vi "SCTL Sector Accumulation Pipelined V2.vi"() -> (3 "New Data?":bool)   [LabVIEW 2013]
uses:
  <vilib>/rvi/FIFO/Fifo_Resource/nirvififoEmulationReadFpgaImpl.vi
  <vilib>/rvi/DataTransferAndStorage/Container/Common/niFpgaContainerGetUniqueNameForEmu.vi
  <vilib>/rvi/Memory/Memory_Emulation/nirvimemoryFastEmulationFpgaImpl.vi
  <instcachedir>/0/nirvimemoryFastEmulationFpgaImpl_5FBAB50466BC4C939F684F8805638BFC.lvgen/nirvimemoryFastEmulationFpgaImpl_5FBAB50466BC4C939F684F8805638BFC_011.vi
  <vilib>/rvi/Memory/Memory_Emulation/nirvimemoryFastEmulation.vi
  <vilib>/rvi/Memory/Memory_Emulation/nirvimemoryEmulation.vi
  <vilib>/rvi/DataTransferAndStorage/Container/XNode/niFpgaContainer.xnode
  <vilib>/rvi/FIFO/Fifo_Resource/nirvififoEmulationRead.vi
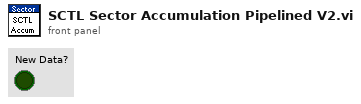
[diagram p1: front panel]
types:
  T1 = cluster{"Accumulated Intensity":u32, "Count":u16}
  T2 = cluster{"Accumulated Intensity":u32, "Count":u16}[]
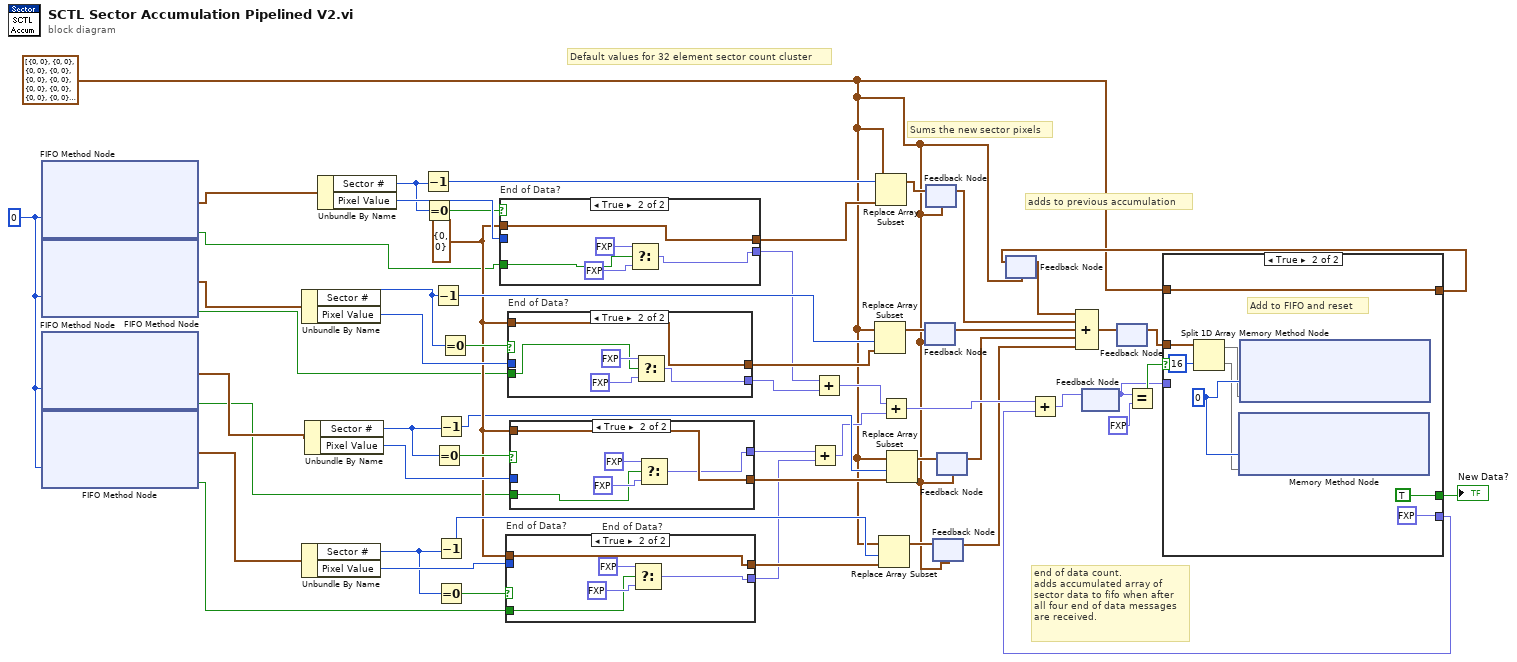
[diagram p0: block diagram]
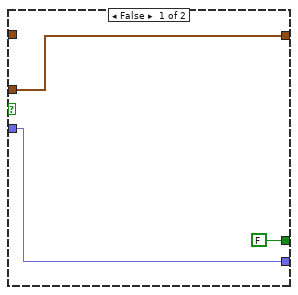
[diagram p2: hidden frame]
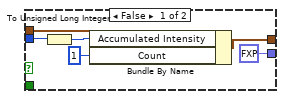
[diagram p3: hidden frame]
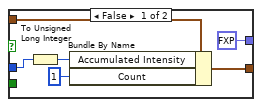
[diagram p4: hidden frame]
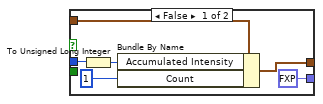
[diagram p5: hidden frame]
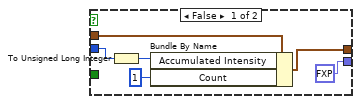
[diagram p6: hidden frame]
diagram:
  w32 = T1 {"Accumulated Intensity"=0, "Count"=0} ("Accumulated Sector Cluster")
  w1 = T2 [{"Accumulated Intensity"=0, "Count"=0}, {"Accumulated Intensity"=0, "Count"=0}, {"Accumulated Intensity"=0, "Count"=0}, {"Accumulated Intensity"=0, "Count"=0}, {"Accumulated Intensity"=0, "Count"=0}, {"Accumulated Intensity"=0, "Count"=0}, {"Accumulated Intensity"=0, "Count"=0}, {"Accumulated Intensity"=0, "Count"=0}, {"Accumulated Intensity"=0, "Count"=0}, {"Accumulated Intensity"=0, "Count"=0}, {"Accumulated Intensity"=0, "Count"=0}, {"Accumulated Intensity"=0, "Count"=0}, {"Accumulated Intensity"=0, "Count"=0}, {"Accumulated Intensity"=0, "Count"=0}, {"Accumulated Intensity"=0, "Count"=0}, {"Accumulated Intensity"=0, "Count"=0}, {"Accumulated Intensity"=0, "Count"=0}, {"Accumulated Intensity"=0, "Count"=0}, {"Accumulated Intensity"=0, "Count"=0}, {"Accumulated Intensity"=0, "Count"=0}, {"Accumulated Intensity"=0, "Count"=0}, {"Accumulated Intensity"=0, "Count"=0}, {"Accumulated Intensity"=0, "Count"=0}, {"Accumulated Intensity"=0, "Count"=0}, {"Accumulated Intensity"=0, "Count"=0}, {"Accumulated Intensity"=0, "Count"=0}, {"Accumulated Intensity"=0, "Count"=0}, {"Accumulated Intensity"=0, "Count"=0}, {"Accumulated Intensity"=0, "Count"=0}, {"Accumulated Intensity"=0, "Count"=0}, {"Accumulated Intensity"=0, "Count"=0}, {"Accumulated Intensity"=0, "Count"=0}] ("Data")
  w56 = 0 ("Timeout")
  # "end of data count.\nadds accumulated array of\nsector data to fifo when after\nall four end of data messages\nare received."
  # "adds to previous accumulation"
  # "Sums the new sector pixels"
  # "Default values for 32 element sector count cluster"
  n1 = xnode ("FIFO Method Node")("Timeout"=w56) -> ("Element"=w28:cluster{"Sector #":u8, "Pixel Value":u8}, "Timed Out?"=w24:bool)  [unwired: 1 in, 1 out]
  n2 = xnode ("FIFO Method Node")("Timeout"=w56) -> ("Element"=w27:cluster{"Sector #":u8, "Pixel Value":u8}, "Timed Out?"=w23:bool)  [unwired: 1 in, 1 out]
  n3 = xnode ("FIFO Method Node")("Timeout"=w56) -> ("Element"=w26:cluster{"Sector #":u8, "Pixel Value":u8}, "Timed Out?"=w22:bool)  [unwired: 1 in, 1 out]
  n4 = xnode ("FIFO Method Node")("Timeout"=w56) -> ("Element"=w25:cluster{"Sector #":u8, "Pixel Value":u8}, "Timed Out?"=w21:bool)  [unwired: 1 in, 1 out]
  n5 = Unbundle By Name(w27) -> ("Sector #"=w42:u8, "Pixel Value"=w52:u8)
  n6 = Unbundle By Name(w25) -> ("Sector #"=w38:u8, "Pixel Value"=w46:u8)
  n7 = Unbundle By Name(w26) -> ("Sector #"=w40:u8, "Pixel Value"=w49:u8)
  n8 = Unbundle By Name(w28) -> ("Sector #"=w44:u8, "Pixel Value"=w54:u8)
  n9 = Decrement(x=w44) -> (x-1=w55:u8)
  n10 = Equal To 0?(x=w44) -> (x = 0?=w43:bool)
  n11 = Decrement(x=w42) -> (x-1=w51:u8)
  n12 = Equal To 0?(x=w40) -> (x = 0?=w39:bool)
  n13 = Decrement(x=w40) -> (x-1=w30:u8)
  n14 = Decrement(x=w38) -> (x-1=w48:u8)
  n15 = Equal To 0?(x=w38) -> (x = 0?=w37:bool)
  n16 = Equal To 0?(x=w42) -> (x = 0?=w41:bool)
  n17 = case "End of Data?" shown="True" w43 {
    tunnel: w54 -> [w58 _]
    tunnel: [w62 w67] -> w53
    tunnel: w32 -> [w61 w67]
    tunnel: [fxp<+,1,1> 0.0 w63] -> w20
    tunnel: w24 -> [_ w66]
    frame False {
      n18 = To Unsigned Long Integer(number=w58) -> (unsigned 32bit integer=w57:u32)
      n19 = Bundle By Name(cluster=w61, "Accumulated Intensity"=w57, "Count"=u16 1) -> (w62:T1)
    }
    frame True {
      n20 = Select(t=fxp<+,1,1> 0.0, s=w66, f=fxp<+,1,1> 1.0) -> (s? t:f=w63:fxp<+,1,1>)
    }
  }
  n21 = case "End of Data?" shown="True" w37 {
    tunnel: [w73 w78] -> w47
    tunnel: w32 -> [w72 w78]
    tunnel: w46 -> [w69 _]
    tunnel: [fxp<+,1,1> 0.0 w74] -> w17
    tunnel: w21 -> [_ w75]
    frame False {
      n22 = To Unsigned Long Integer(number=w69) -> (unsigned 32bit integer=w68:u32)
      n23 = Bundle By Name(cluster=w72, "Accumulated Intensity"=w68, "Count"=u16 1) -> (w73:T1)
    }
    frame True {
      n24 = Select(t=fxp<+,1,1> 0.0, s=w75, f=fxp<+,1,1> 1.0) -> (s? t:f=w74:fxp<+,1,1>)
    }
  }
  n25 = case "End of Data?" shown="True" w41 {
    tunnel: w52 -> [w80 _]
    tunnel: w32 -> [w84 w89]
    tunnel: [w83 w89] -> w45
    tunnel: [fxp<+,1,1> 0.0 w85] -> w19
    tunnel: w23 -> [_ w86]
    frame False {
      n26 = To Unsigned Long Integer(number=w80) -> (unsigned 32bit integer=w79:u32)
      n27 = Bundle By Name(cluster=w84, "Accumulated Intensity"=w79, "Count"=u16 1) -> (w83:T1)
    }
    frame True {
      n28 = Select(t=fxp<+,1,1> 0.0, s=w86, f=fxp<+,1,1> 1.0) -> (s? t:f=w85:fxp<+,1,1>)
    }
  }
  n29 = case "End of Data?" shown="True" w39 {
    tunnel: [w95 w100] -> w50
    tunnel: w49 -> [w91 _]
    tunnel: w32 -> [w94 w100]
    tunnel: [fxp<+,1,1> 0.0 w96] -> w18
    tunnel: w22 -> [_ w97]
    frame False {
      n30 = To Unsigned Long Integer(number=w91) -> (unsigned 32bit integer=w90:u32)
      n31 = Bundle By Name(cluster=w94, "Accumulated Intensity"=w90, "Count"=u16 1) -> (w95:T1)
    }
    frame True {
      n32 = Select(t=fxp<+,1,1> 0.0, s=w97, f=fxp<+,1,1> 1.0) -> (s? t:f=w96:fxp<+,1,1>)
    }
  }
  n33 = Add(x=w18, y=w17) -> (x+y=w15:fxp<+,2,2>)
  n34 = Add(x=w20, y=w19) -> (x+y=w16:fxp<+,2,2>)
  n35 = Replace Array Subset(array=w1, new element=w45, index=w51) -> (w7:T2)
  n36 = Replace Array Subset(array=w1, new element=w53, index=w55) -> (w9:T2)
  n37 = Replace Array Subset(array=w1, new element=w47, index=w48) -> (w3:T2)
  n38 = Add(x=w16, y=w15) -> (x+y=w14:fxp<+,3,3>)
  n39 = Replace Array Subset(array=w1, new element=w50, index=w30) -> (w6:T2)
  n40 = feedback #1(w1) -> (w5:T2)
  n41 = feedback-in #1(w7) -> ()
  n42 = feedback #2(w1) -> (w8:T2)
  n43 = feedback-in #2(w9) -> ()
  n44 = feedback #3(w1) -> (w2:T2)
  n45 = feedback-in #3(w3) -> ()
  n46 = feedback #4(w1) -> (w4:T2)
  n47 = feedback-in #4(w6) -> ()
  n48 = feedback #5(w1) -> (w29:T2)
  n49 = Compound Arithmetic op=ADD(w29, w8, w5, w4, w2) -> (w11:T2)
  n50 = feedback #6() -> (w34:fxp<+,3,3>)  [unwired: 1 in]
  n51 = feedback #7() -> (w10:T2)  [unwired: 1 in]
  n52 = feedback-in #7(w11) -> ()
  n53 = Equal?(x=w34, y=fxp<+,3,3> 4.0) -> (x = y?=w35:bool)
  n54 = case shown="True" w35 {
    tunnel: w10 -> [w103 w108]
    tunnel: [w101 fxp<+,3,3> 0.0] -> w13
    tunnel: w34 -> [w101 _]
    tunnel: [w103 w110] -> w33
    tunnel: w1 -> [_ w110]
    tunnel: [FALSE ("New Data?") TRUE ("New Data?")] -> w31
    frame False {
    }
    frame True {
      w109 = 0 ("Timeout")
      # "Add to FIFO and reset"
      n55 = Split 1D Array(array=w108, index=16) -> (first subarray=w106:T2, second subarray=w105:T2)
      n56 = xnode ("Memory Method Node")("Address"=w109, "Data"=w105) -> ()  [unwired: 1 in, 1 out]
      n57 = xnode ("Memory Method Node")("Address"=w109, "Data"=w106) -> ()  [unwired: 1 in, 1 out]
    }
  }
  "New Data?" <- w31
  n58 = feedback-in #5(w33) -> ()
  n59 = Add(x=w14, y=w13) -> (x+y=w12:fxp<+,3,3>)
  n60 = feedback-in #6(w12) -> ()
